vi "Read_Data.vi"(8 "error in":errorcluster, 9 "Shift_Register_In":i16[](array[numeric]), 11 "FPGA VI Reference In":T1) -> (0 "error out":errorcluster, 1 "Shift_Register_Out":i16[](array[numeric]), 3 "FPGA VI Reference Out 2":T2)   [LabVIEW 2025]
uses:
  FPGA_ref_out.ctl
  FPGA_ref_in.ctl
  <vilib>/Utility/error.llb/Error Cluster From Error Code.vi
  <vilib>/rvi/errors/niLvFpgaAdjustHostInterfaceError.vi
  <vilib>/rvi/interface/nirviMethod/nirviMethod.xnode
  <vilib>/FPGAPlugInAG/Dynamic/niLvFpga_ReadFifo_Dynamic.vi
  <vilib>/rvi/errors/niLvFpgaMergeErrorWithErrorCode.vi
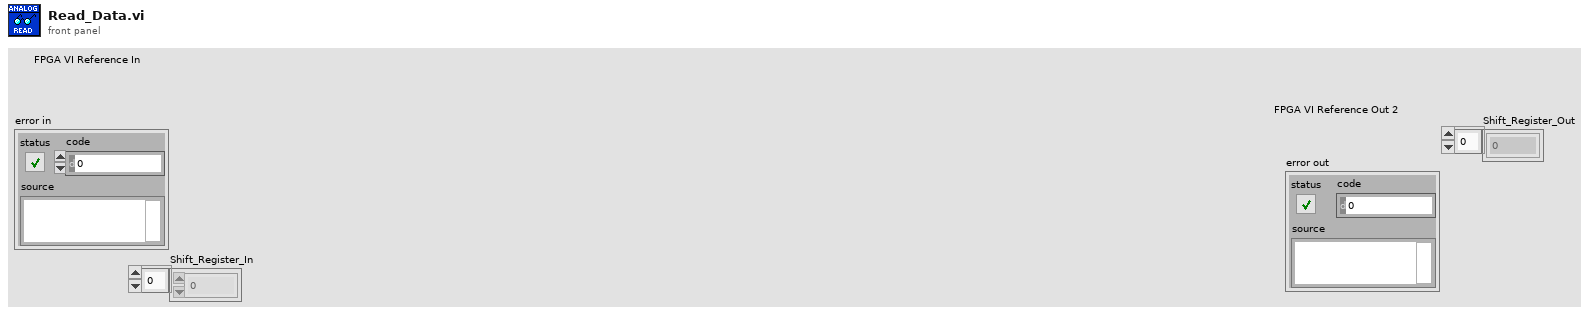
[diagram p1: front panel]
types:
  T1 = typedef "FPGA_ref_in.ctl" = refnum<k20>
  T2 = typedef "FPGA_ref_out.ctl" = refnum<k20>
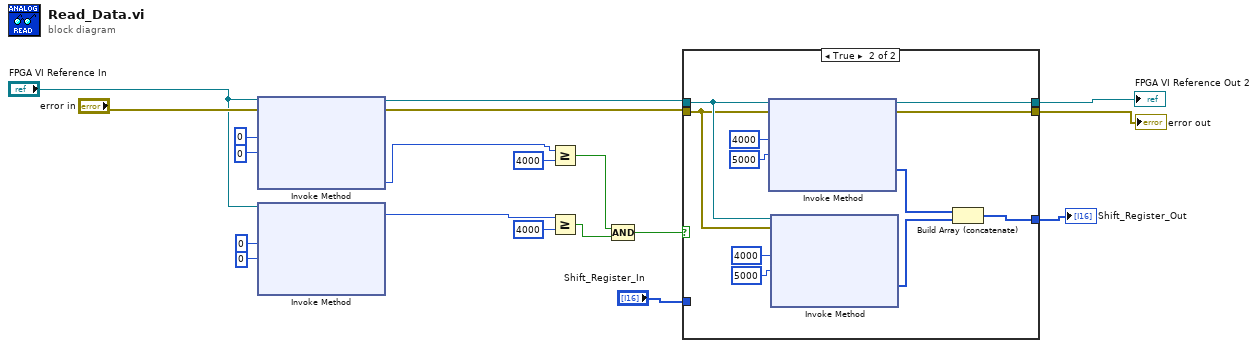
[diagram p0: block diagram]
diagram:
  n1 = xnode "Invoke Method"("FPGA VI Reference In"="FPGA VI Reference In", "error in"="error in", "Number of Elements"=u32 0, "Timeout (ms)"=0) -> ("FPGA VI Reference Out"=w16:T1, "error out"=w15:errorcluster, "Elements Remaining"=w1:u32)  [unwired: 1 out]
  n2 = xnode "Invoke Method"("FPGA VI Reference In"="FPGA VI Reference In", "Number of Elements"=u32 0, "Timeout (ms)"=0) -> ("Elements Remaining"=w11:u32)  [unwired: 1 in, 3 out]
  n3 = Greater Or Equal?(x=w1, y=u32 4000) -> (x >= y?=w10:bool)
  n4 = Greater Or Equal?(x=w11, y=u32 4000) -> (x >= y?=w9:bool)
  n5 = Compound Arithmetic op=AND(w10, w9) -> (w8:bool)
  n6 = case shown="True" w8 {
    tunnel: [w22 w25] -> w2
    tunnel: [w21 w26] -> w5
    tunnel: w16 -> [w22 w29]
    tunnel: w15 -> [w21 w28]
    tunnel: [w20 w23] -> w7
    tunnel: "Shift_Register_In" -> [w20 _]
    frame False {
    }
    frame True {
      n7 = xnode "Invoke Method"("FPGA VI Reference In"=w29, "error in"=w28, "Number of Elements"=u32 4000, "Timeout (ms)"=5000) -> ("FPGA VI Reference Out"=w25:T1, "error out"=w26:errorcluster, "Data"=w24:i16[])  [unwired: 1 out]
      n8 = xnode "Invoke Method"("FPGA VI Reference In"=w29, "error in"=w28, "Number of Elements"=u32 4000, "Timeout (ms)"=5000) -> ("Data"=w27:i16[])  [unwired: 3 out]
      n9 = Build Array (concatenate)(w24, w27) -> (w23:i16[])
    }
  }
  "error out" <- w5
  "Shift_Register_Out" <- w7
  "FPGA VI Reference Out 2" <- w2
